vi "Get Error Description.vi"(10 "Code":u8) -> (2 "STP Error":T1)   [LabVIEW 2023, in "HardwareAbstractionLayer_LVOOP.lvlib" / "CAN Application Protocols Lib.lvlib" / "STP Protocol.lvclass"]
uses:
  STP Protocol.lvclass
  Ctrls/STP Error Cluster.ctl
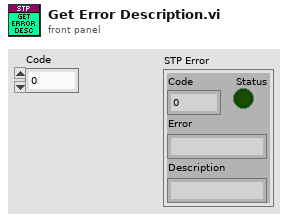
[diagram p1: front panel]
types:
  T1 = typedef "HardwareAbstractionLayer_LVOOP.lvlib/CAN Application Protocols Lib.lvlib/STP Protocol.lvclass/STP Error Cluster.ctl" = cluster{"Status":bool, "Code":u8, "Error":string, "Description":string}
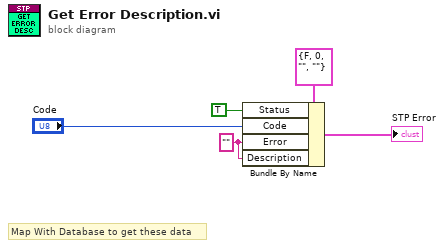
[diagram p0: block diagram]
diagram:
  w1 = "" ("Error")
  # "Map With Database to get these data"
  n1 = Bundle By Name(cluster=T1 {"Status"=FALSE, "Code"=0, "Error"="", "Description"=""} ("STP Error"), "Status"=TRUE ("Error"), "Code"="Code", "Error"=w1, "Description"=w1) -> (→"STP Error":T1)
